vi "Show_virtual variables.vi"() -> ()   [LabVIEW 2022 SP3]
panel:
  out "Signals_value_string":string[](array[string])
  out "Signals_value_Array":dbl[](array[numeric])
  out "Signals_name":string[](array[string])
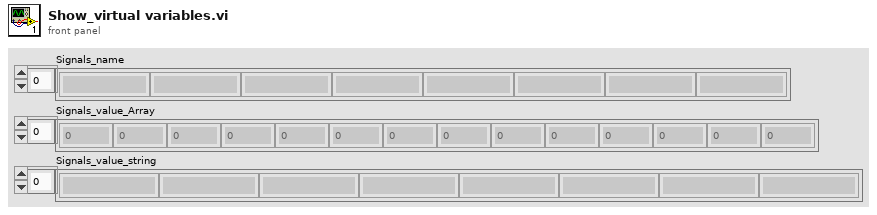
[diagram p1: front panel]
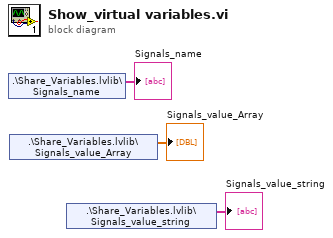
[diagram p0: block diagram]
diagram:
  n1 = shared-variable ".\\Share_Variables.lvlib\\Signals_name"() -> (→"Signals_name":string[])  [unwired: 1 in, 1 out]
  n2 = shared-variable ".\\Share_Variables.lvlib\\Signals_value_Array"() -> (→"Signals_value_Array":dbl[])  [unwired: 1 in, 1 out]
  n3 = shared-variable ".\\Share_Variables.lvlib\\Signals_value_string"() -> (→"Signals_value_string":string[])  [unwired: 1 in, 1 out]
